vi "T7.vi"() -> ()   [LabVIEW 2020]
panel:
  in  "A":dbl
  out "Boolean":bool
  out "Boolean":bool
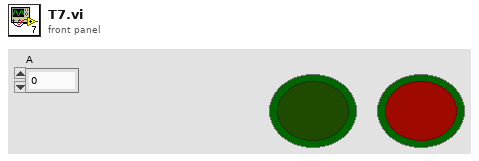
[diagram p1: front panel]
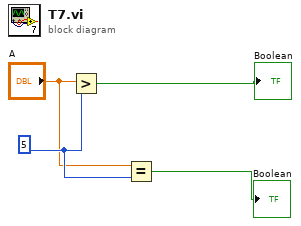
[diagram p0: block diagram]
diagram:
  w3 = 5
  n1 = Greater?(x="A", y=w3) -> (0:→"Boolean":bool)
  n2 = Equal?(x="A", y=w3) -> (x = y?=→"Boolean":bool)
